vi "Fridge_Valve_Main.vi"(7 "stop_external":refnum<vi>, 8 "cluster_ref_fridge_valve":T1) -> ()   [LabVIEW 2019]
uses:
  cluster_ref_fridge_valve.ctl
  C:/Program Files/National Instruments/LabVIEW 2019/vi.lib/ULx/ULx_LV.dll
  Program Files/National Instruments/LabVIEW 2019/vi.lib/ULx/ULx_LV.dll
panel:
  in  "Logging":bool=TRUE
  out "b.v.m. alarm":u16
  out "r.v.m. alarm":u16
  out "b.v.m. status":u16
  out "r.v.m. status":u16
  out "B.V. Opening Slide":dbl(slide) scale=-0.1..3.1 scale format="%.1g"
  out "R.V. Opening Slide":dbl(slide) scale=-0.1..3.1 scale format="%.1f"
  in  "rv_auto_control":bool caption="Automated\nRun-Valve\nControl"
  in  "r.v.m. power":bool=TRUE caption="Motor\nPower"
  in  "Set RV Opening":dbl caption="Set Turns" min=-0.1 max=3.1 step=0.1 format="%.2f"
  out "R.V. Motor Status":bool
  in  "R.V. VISA":refnum<visa-resource-name>="COM29"
  out "He Level":waveform(dbl)[](graph)
  out "He Level":dbl(slide) scale=0.0..100.0
  out "Level Probe Status":bool
  in  "AMI1700 VISA":refnum<visa-resource-name>="COM31"
  in  "Set BV Opening":dbl caption="Set Turns" min=-0.1 max=3.1 step=0.1 format="%.2f"
  out "bv_step_init":i32
  out "rv_step_init":i32
  out "Run Valve Steps":i32 caption="Motor Step"
  out "Run Valve ADC":dbl caption="ADC"
  out "Bypass Valve ADC":dbl caption="ADC"
  out "Bypass Valve Step":i32 caption="Motor Step"
  out "Bypass Valve Turns":waveform(dbl)[](graph)
  out "Run Valve Turns":waveform(dbl)[](graph)
  out "ADC Status":bool=TRUE
  out "Last Updated":timestamp format="%<%Y-%m-%d %H:%M:%S>T"
  in  "B.V. VISA":refnum<visa-resource-name>="COM21"
  in  "b.v.m. power":bool=TRUE caption="Motor\nPower"
  in  "Stop":bool
  in  "Pause":bool=TRUE
  out "B.V. Motor Status":bool
  in  "Enable Advanced Controls":bool
  # "Fridge Valve Panel"
  # "Level Probe"
  # "Run Valve"
  # "Bypass Valve"
  # "Motor Status"
  # "Motor Alarm"
  # "Initial Steps"
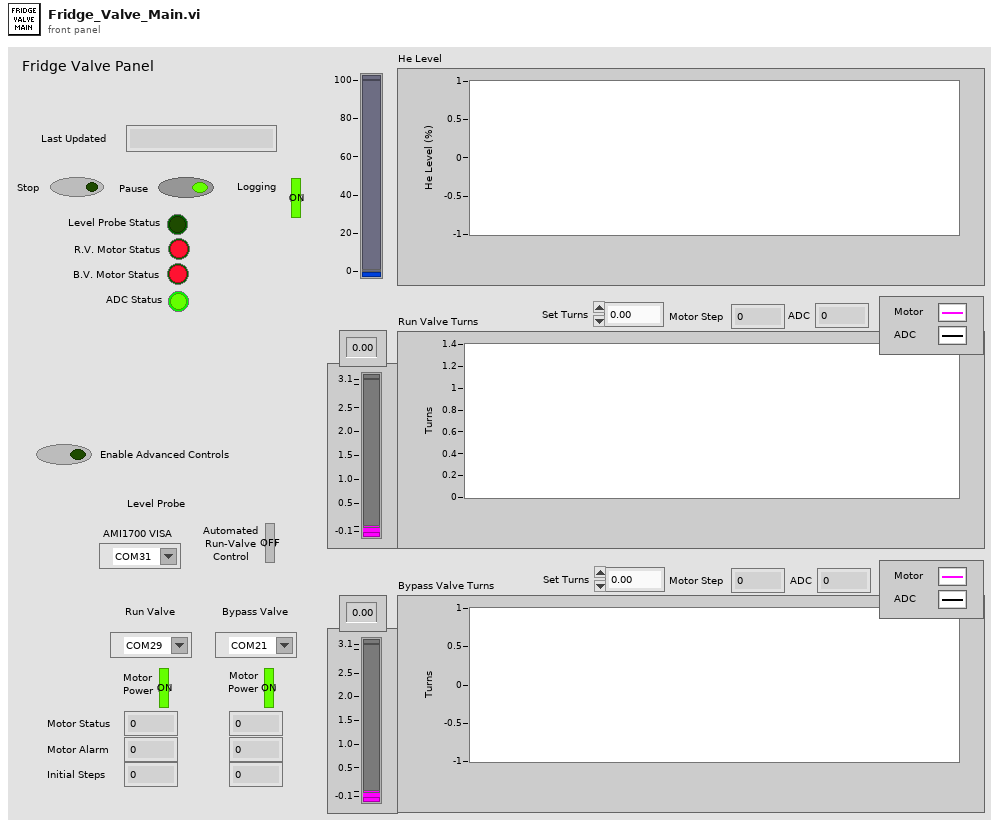
[diagram p1: front panel]
types:
  T1 = typedef "cluster_ref_fridge_valve.ctl" = cluster{"Status":refnum<vi>, "RVO":refnum<vi>, "BVO":refnum<vi>, "He Level":refnum<vi>}
  T2 = enum8{"Enabled", "Disabled", "Disabled and Grayed Out"}
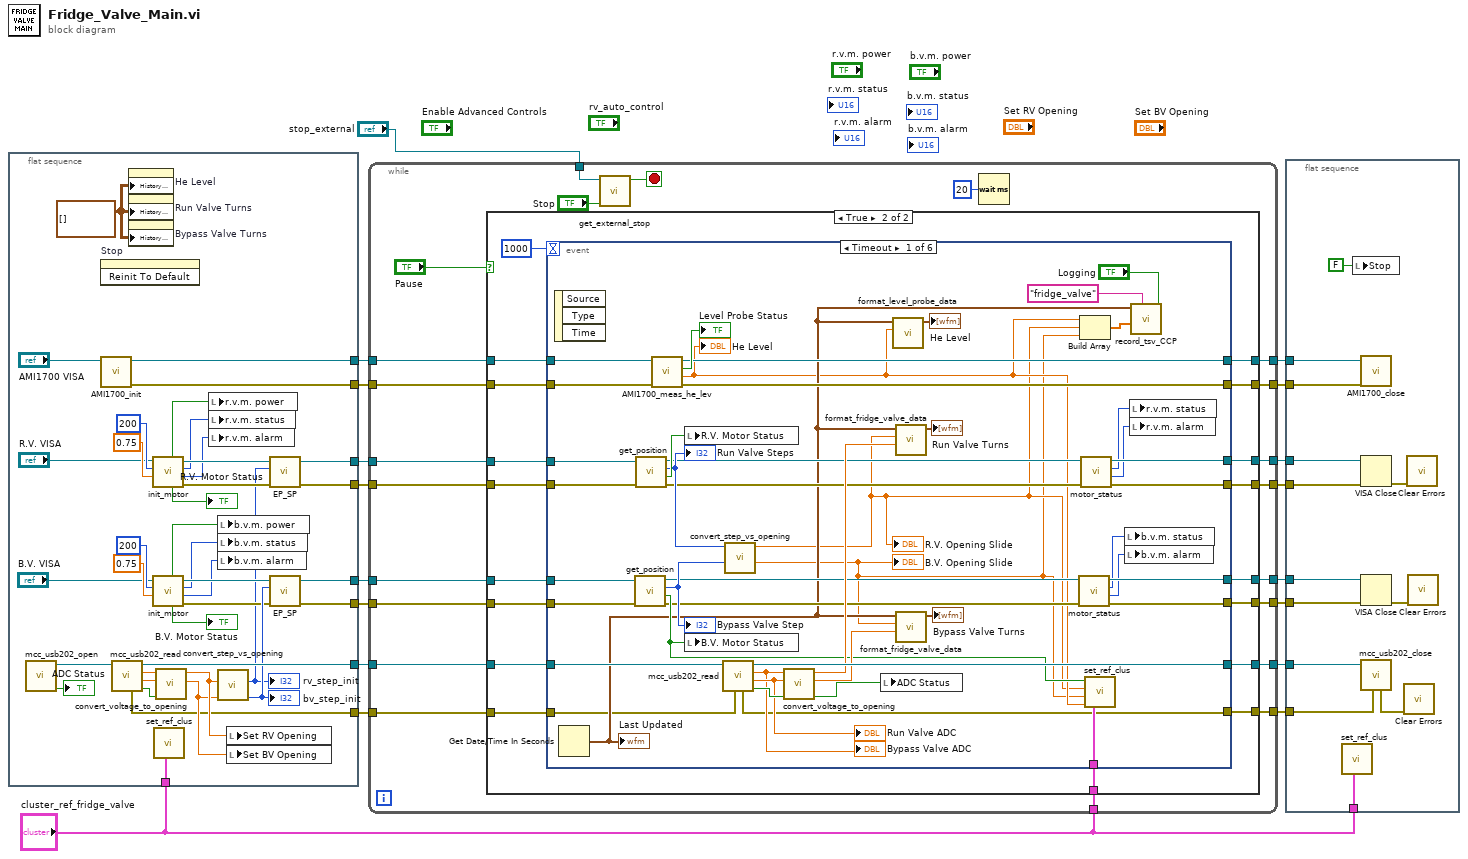
[diagram p0: block diagram]
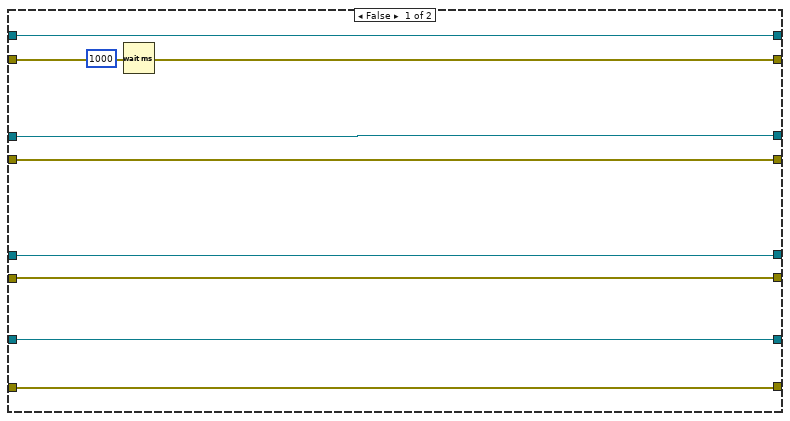
[diagram p2: hidden frame]
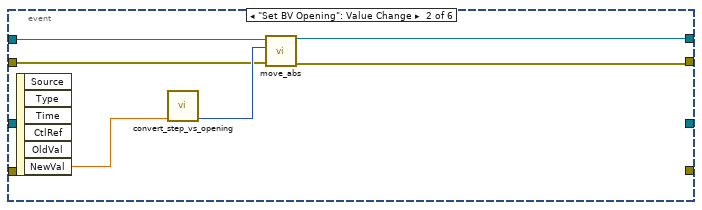
[diagram p3: hidden frame]
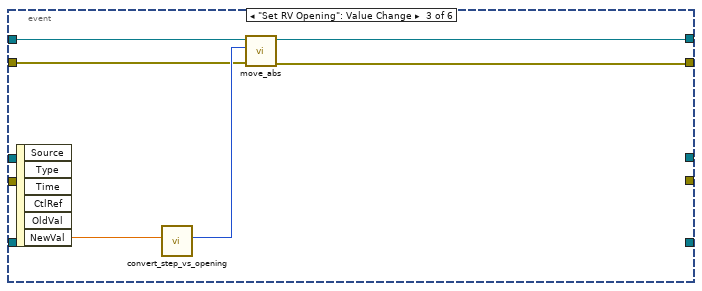
[diagram p4: hidden frame]
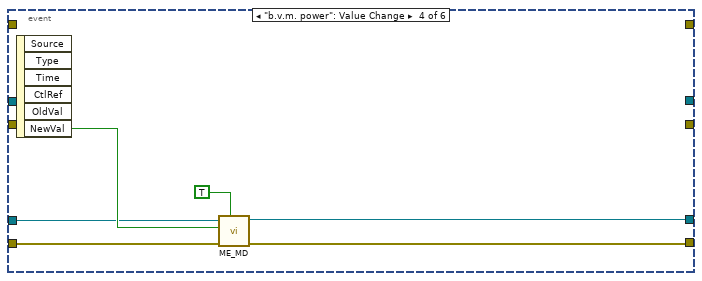
[diagram p5: hidden frame]
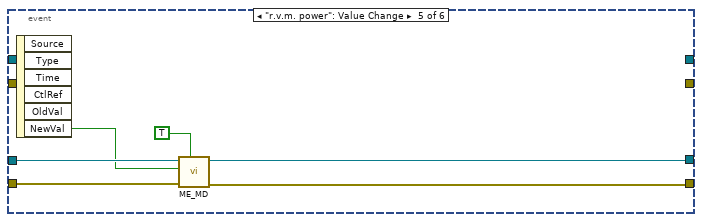
[diagram p6: hidden frame]
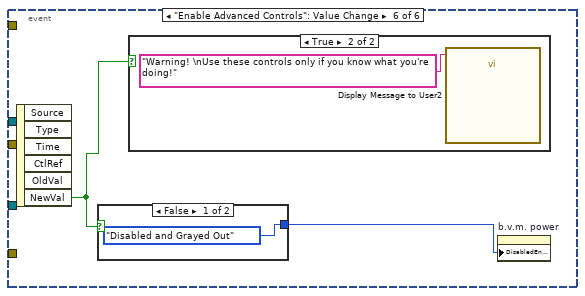
[diagram p7: hidden frame]
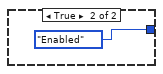
[diagram p8: hidden frame]
diagram:
  n1 = flat-sequence {
    tunnel: [w49] -> w12
    tunnel: [w54] -> w11
    tunnel: [w48] -> w13
    tunnel: [w41] -> w16
    tunnel: [w40] -> w17
    tunnel: [w34] -> w14
    tunnel: [w33] -> w15
    tunnel: "cluster_ref_fridge_valve" -> [w20]
    tunnel: [w19] -> w2
    frame #0 {
      w31 = waveform(dbl)[][] [] ("History Data")
      n2 = call "mcc_usb202_open.vi"() -> ("status"=→"ADC Status":bool, "task out"=w55:refnum<k24>)  [unwired: 9 in, 1 out]
      n3 = invoke on="Stop" class="Bool (strict)" method="Reinit To Default"() -> ()  [unwired: 3 in, 3 out]
      n4 = call "AMI1700_init.vi"("VISA in"="AMI1700 VISA") -> ("error out"=w41:errorcluster, "VISA out"=w40:refnum<visa-resource-name>)  [unwired: 9 in]
      n5 = call "mcc_usb202_read.vi"("task in"=w55) -> ("status"=w51:bool, "V1"=w52:dbl, "V0"=w53:dbl, "task out"=w54:refnum<k24>, "error out"=w19:errorcluster)  [unwired: 6 in]
      n6 = property on="He Level" class="WFChart (strict)"("History Data"=w31) -> ()  [unwired: 2 in, 2 out]
      n7 = property on="Run Valve Turns" class="WFChart (strict)"("History Data"=w31) -> ()  [unwired: 2 in, 2 out]
      n8 = property on="Bypass Valve Turns" class="WFChart (strict)"("History Data"=w31) -> ()  [unwired: 2 in, 2 out]
      n9 = call "init_motor.vi"("velocity"=0.75, "steps_per_rev"=200, "VISA in"="R.V. VISA") -> ("error out"=w36:errorcluster, "motor_alarm"=w22:i32, "motor_status"=w24:i32, "VISA out"=w37:refnum<visa-resource-name>, "status"=→"R.V. Motor Status":bool, "is_on"=w26:bool)  [unwired: 3 in]
      n10 = call "init_motor.vi"("velocity"=0.75, "steps_per_rev"=200, "VISA in"="B.V. VISA") -> ("error out"=w43:errorcluster, "motor_alarm"=w21:i32, "motor_status"=w23:i32, "VISA out"=w44:refnum<visa-resource-name>, "status"=→"B.V. Motor Status":bool, "is_on"=w25:bool)  [unwired: 3 in]
      n11 = call "set_ref_clus.vi"("cluster_ref"=w20) -> ()  [unwired: 11 in]
      n12 = call "convert_voltage_to_opening.vi"("status_in"=w51, "bypass_valve_voltage"=w52, "run_valve_voltage"=w53) -> ("bypass_valve_opening"=w29:dbl, "run_valve_opening"=w30:dbl)  [unwired: 6 in, 1 out]
      n13 = local write "r.v.m. power"(w26) -> ()
      n14 = local write "r.v.m. status"(w24) -> ()
      n15 = local write "r.v.m. alarm"(w22) -> ()
      n16 = local write "b.v.m. power"(w25) -> ()
      n17 = local write "b.v.m. status"(w23) -> ()
      n18 = local write "b.v.m. alarm"(w21) -> ()
      n19 = call "convert_step_vs_opening.vi"("bypass_valve_opening_in"=w29, "run_valve_opening_in"=w30) -> ("bypass_valve_step_out"=w50:i32, "run_valve_step_out"=w32:i32)  [unwired: 6 in, 2 out]
      "rv_step_init" <- w32
      "bv_step_init" <- w50
      n20 = local write "Set RV Opening"(w30) -> ()
      n21 = local write "Set BV Opening"(w29) -> ()
      n22 = call "EP_SP.vi"("error in"=w36, "new_position"=w32, "VISA in"=w37) -> ("error out"=w34:errorcluster, "VISA out"=w33:refnum<visa-resource-name>)  [unwired: 7 in]
      n23 = call "EP_SP.vi"("error in"=w43, "new_position"=w50, "VISA in"=w44) -> ("error out"=w49:errorcluster, "VISA out"=w48:refnum<visa-resource-name>)  [unwired: 7 in]
    }
  }
  n24 = while {
    tunnel: "cluster_ref_fridge_valve" -> [w76]
    tunnel: "stop_external" -> [w59]
    tunnel: w17 -> [w75]
    tunnel: w16 -> [w74]
    tunnel: w15 -> [w73]
    tunnel: w14 -> [w72]
    tunnel: w13 -> [w71]
    tunnel: w12 -> [w70]
    tunnel: w11 -> [w69]
    tunnel: [w68] -> w10
    tunnel: [w67] -> w9
    tunnel: [w66] -> w8
    tunnel: [w65] -> w7
    tunnel: [w64] -> w6
    tunnel: [w63] -> w5
    tunnel: [w62] -> w4
    tunnel: w2 -> [w58]
    tunnel: [w57] -> w1
    stop <- w61 stop-if-true
    n25 = case shown="True" "Pause" {
      tunnel: w76 -> [_ w105]
      tunnel: w75 -> [w87 w104]
      tunnel: w74 -> [w86 w103]
      tunnel: w73 -> [w85 w102]
      tunnel: w72 -> [w84 w101]
      tunnel: w71 -> [w83 w100]
      tunnel: w70 -> [w82 w99]
      tunnel: w69 -> [w81 w98]
      tunnel: [w82 w96] -> w68
      tunnel: [w83 w95] -> w67
      tunnel: [w86 w94] -> w66
      tunnel: [w87 w93] -> w65
      tunnel: [w84 w92] -> w64
      tunnel: [w85 w91] -> w63
      tunnel: [w81 w90] -> w62
      tunnel: w58 -> [w79 w89]
      tunnel: [w79 w88] -> w57
      frame False {
        n26 = Wait (ms)(milliseconds to wait=u32 1000) -> ()  [unwired: 1 out]
      }
      frame True {
        n27 = event shown="[0] Timeout" {
          selector: _ -> [_ _ _ _ _ _]
          dyn-events: _ -> [_ _ _ _ _ _]
          timeout: 1000 -> [_ _ _ _ _ _]
          tunnel: w100 -> [w141 w156 _ w167 _ _]
          tunnel: w99 -> [w140 w154 _ w168 _ _]
          tunnel: w98 -> [w151 _ _ _ _ _]
          tunnel: [w149 _ _ _ _ _] -> w90
          tunnel: w105 -> [w138 _ _ _ _ _]
          tunnel: w103 -> [w135 _ _ _ _ _]
          tunnel: w104 -> [w134 _ _ _ _ _]
          tunnel: w101 -> [w132 _ w160 _ w174 _]
          tunnel: w102 -> [w131 _ w161 _ w175 _]
          tunnel: [w128 _ _ _ _ _] -> w93
          tunnel: [w127 _ _ _ _ _] -> w94
          tunnel: [w119 w153 _ w166 _ _] -> w95
          tunnel: [w118 w152 _ w165 _ _] -> w96
          tunnel: [w125 _ w159 _ w172 _] -> w91
          tunnel: [w124 _ w158 _ w173 _] -> w92
          tunnel: w89 -> [w107 _ _ _ _ _]
          tunnel: [w106 _ _ _ _ _] -> w88
          event Timeout {
            n28 = event-data() -> ()  [unwired: 1 in, 3 out]
            n29 = Get Date/Time In Seconds() -> (seconds since 1Jan1904=w114:timestamp)
            "Last Updated" <- w114
            n30 = call "get_position.vi"("error in"=w140, "VISA"=w141) -> ("error out"=w117:errorcluster, "status"=w137:bool, "Position"=w139:i32, "VISA out"=w126:refnum<visa-resource-name>)  [unwired: 6 in]
            "Bypass Valve Step" <- w139
            n31 = call "get_position.vi"("error in"=w132, "VISA"=w131) -> ("error out"=w122:errorcluster, "status"=w130:bool, "Position"=w129:i32, "VISA out"=w123:refnum<visa-resource-name>)  [unwired: 6 in]
            "Run Valve Steps" <- w129
            n32 = call "AMI1700_meas_he_lev.vi"("error in"=w135, "VISA in"=w134) -> ("error out"=w127:errorcluster, "level"=w110:dbl, "status"=→"Level Probe Status":bool, "VISA out"=w128:refnum<visa-resource-name>)  [unwired: 6 in]
            "He Level" <- w110
            n33 = local write "R.V. Motor Status"(w130) -> ()
            n34 = local write "B.V. Motor Status"(w137) -> ()
            n35 = call "mcc_usb202_read.vi"("error in"=w107, "task in"=w151) -> ("status"=w150:bool, "V1"=w144:dbl, "V0"=w143:dbl, "task out"=w149:refnum<k24>, "error out"=w106:errorcluster)  [unwired: 5 in]
            "Bypass Valve ADC" <- w144
            "Run Valve ADC" <- w143
            n36 = call "convert_step_vs_opening.vi"("bypass_valve_step_in"=w139, "run_valve_step_in"=w129) -> ("bypass_valve_opening_out"=w108:dbl, "run_valve_opening_out"=w109:dbl)  [unwired: 6 in, 2 out]
            "R.V. Opening Slide" <- w109
            "B.V. Opening Slide" <- w108
            n37 = call "convert_voltage_to_opening.vi"("status_in"=w150, "bypass_valve_voltage"=w144, "run_valve_voltage"=w143) -> ("status_out"=w142:bool, "bypass_valve_opening"=w147:dbl, "run_valve_opening"=w145:dbl)  [unwired: 6 in]
            n38 = local write "ADC Status"(w142) -> ()
            n39 = call "format_level_probe_data.vi"("he_level"=w110, "time"=w114) -> ("waveform_array"=→"He Level":waveform(dbl)[])  [unwired: 9 in]
            n40 = call "format_fridge_valve_data.vi"("value_adc"=w145, "value_motor"=w109, "time"=w114) -> ("waveform_array"=→"Run Valve Turns":waveform(dbl)[])  [unwired: 8 in]
            n41 = call "format_fridge_valve_data.vi"("value_adc"=w147, "value_motor"=w108, "time"=w114) -> ("waveform_array"=→"Bypass Valve Turns":waveform(dbl)[])  [unwired: 8 in]
            n42 = call "motor_status.vi"("error in"=w117, "VISA"=w126) -> ("error out"=w118:errorcluster, "motor_alarm"=w115:i32, "motor_status"=w116:i32, "VISA out"=w119:refnum<visa-resource-name>)  [unwired: 4 in, 2 out]
            n43 = Build Array(w110, w109, w108) -> (w111:dbl[])
            n44 = call "motor_status.vi"("error in"=w122, "VISA"=w123) -> ("error out"=w124:errorcluster, "motor_alarm"=w120:i32, "motor_status"=w121:i32, "VISA out"=w125:refnum<visa-resource-name>)  [unwired: 4 in, 2 out]
            n45 = call "set_ref_clus.vi"("cluster_ref"=w138, "he_level"=w110, "bypass_valve_opening"=w108, "run_valve_opening"=w109, "status"=w137) -> ()  [unwired: 7 in]
            n46 = local write "b.v.m. status"(w116) -> ()
            n47 = local write "b.v.m. alarm"(w115) -> ()
            n48 = local write "r.v.m. status"(w121) -> ()
            n49 = local write "r.v.m. alarm"(w120) -> ()
            n50 = call "record_tsv_CCP.vi"("logging_on"="Logging", "folder_name"="fridge_valve", "value_array"=w111, "time"=w114) -> ()  [unwired: 6 in, 2 out]
          }
          event "Set BV Opening": Value Change {
            n51 = event-data() -> ("NewVal"=w157:dbl)  [unwired: 1 in, 5 out]
            n52 = call "convert_step_vs_opening.vi"("bypass_valve_opening_in"=w157) -> ("bypass_valve_step_out"=w155:i32)  [unwired: 7 in, 3 out]
            n53 = call "move_abs.vi"("error in"=w154, "Position Aboslute"=w155, "VISA in"=w156) -> ("error out"=w152:errorcluster, "VISA out"=w153:refnum<visa-resource-name>)  [unwired: 7 in]
          }
          event "Set RV Opening": Value Change {
            n54 = event-data() -> ("NewVal"=w163:dbl)  [unwired: 1 in, 5 out]
            n55 = call "convert_step_vs_opening.vi"("run_valve_opening_in"=w163) -> ("run_valve_step_out"=w162:i32)  [unwired: 7 in, 3 out]
            n56 = call "move_abs.vi"("error in"=w160, "Position Aboslute"=w162, "VISA in"=w161) -> ("error out"=w158:errorcluster, "VISA out"=w159:refnum<visa-resource-name>)  [unwired: 7 in]
          }
          event "b.v.m. power": Value Change {
            n57 = event-data() -> ("NewVal"=w169:bool)  [unwired: 1 in, 5 out]
            n58 = call "ME_MD.vi"("do_reset"=TRUE, "error in"=w168, "enable_or_disable"=w169, "VISA in"=w167) -> ("error out"=w165:errorcluster, "VISA out"=w166:refnum<visa-resource-name>)  [unwired: 5 in, 1 out]
          }
          event "r.v.m. power": Value Change {
            n59 = event-data() -> ("NewVal"=w171:bool)  [unwired: 1 in, 5 out]
            n60 = call "ME_MD.vi"("do_reset"=TRUE, "error in"=w174, "enable_or_disable"=w171, "VISA in"=w175) -> ("error out"=w173:errorcluster, "VISA out"=w172:refnum<visa-resource-name>)  [unwired: 5 in, 1 out]
          }
          event "Enable Advanced Controls": Value Change {
            n61 = event-data() -> ("NewVal"=w177:bool)  [unwired: 1 in, 5 out]
            n62 = case shown="False" w177 {
              tunnel: [T2."Disabled and Grayed Out" ("Disabled") T2."Enabled" ("Disabled")] -> w176
              frame False {
              }
              frame True {
              }
            }
            n63 = case shown="True" w177 {
              frame False {
              }
              frame True {
                n64 = call "Display Message to User2"("Message"="Warning! \nUse these controls only if you know what you're doing!") -> ()  [unwired: 9 in, 2 out]
              }
            }
            n65 = property on="b.v.m. power" class="Bool (strict)"("DisabledEnum"=w176) -> ()  [unwired: 2 in, 2 out]
          }
        }
      }
    }
    n66 = call "get_external_stop.vi"("stop_internal"="Stop", "ref_stop_external"=w59) -> ("stop_output"=w61:bool)  [unwired: 9 in]
    n67 = Wait (ms)(milliseconds to wait=u32 20) -> ()  [unwired: 1 out]
  }
  n68 = flat-sequence {
    tunnel: w10 -> [w193]
    tunnel: w9 -> [w192]
    tunnel: w8 -> [w191]
    tunnel: w7 -> [w190]
    tunnel: w6 -> [w189]
    tunnel: w5 -> [w188]
    tunnel: w4 -> [w187]
    tunnel: "cluster_ref_fridge_valve" -> [w186]
    tunnel: w1 -> [w184]
    frame #0 {
      n69 = call "set_ref_clus.vi"("cluster_ref"=w186) -> ()  [unwired: 11 in]
      n70 = local write "Stop"(FALSE ("Stop")) -> ()
      n71 = call "AMI1700_close.vi"("error in"=w191, "VISA in"=w190) -> ()  [unwired: 9 in, 1 out]
      n72 = VISA Close(VISA resource name=w188, error in (no error)=w189) -> (error out=w183:errorcluster)
      n73 = VISA Close(VISA resource name=w192, error in (no error)=w193) -> (error out=w182:errorcluster)
      n74 = call "mcc_usb202_close.vi"("error in"=w184, "task in"=w187) -> ("error out"=w181:errorcluster)  [unwired: 8 in, 1 out]
      n75 = call <vilib>:"Clear Errors.vi"("error in (no error)"=w181) -> ()  [unwired: 5 in, 2 out]
      n76 = call <vilib>:"Clear Errors.vi"("error in (no error)"=w183) -> ()  [unwired: 5 in, 2 out]
      n77 = call <vilib>:"Clear Errors.vi"("error in (no error)"=w182) -> ()  [unwired: 5 in, 2 out]
    }
  }
